vi "Create Key Map Primitive.vi"(8 "error in (no error)":errorcluster, 10 "Tresholds":refnum<class "1D Array s32.lvclass">, 11 "Keys":refnum<class "2D Array u32.lvclass">) -> (0 "error out":errorcluster, 2 "Transposed Key MapPrimitive":refnum<class "2D Array u32.lvclass">, 3 "Key Map Primitive":refnum<class "2D Array u32.lvclass">)   [LabVIEW 2020, in "G2CPU Line Profile.lvlib"]
uses:
  G2CPU Line Profile.lvlib
  <vilib>/Natan Biesmans/G2CPU GPU and CPU HPC Toolkit/G2CPU Libraries/Arrays/2DArray/u32/2D Array u32.lvclass
  C:/Program Files/National Instruments/LabVIEW 2025/vi.lib/Natan Biesmans/G2CPU GPU and CPU HPC Toolkit/G2CPU Libraries/Arrays/Array/Array Prototype.lvclass
  <vilib>/Natan Biesmans/G2CPU GPU and CPU HPC Toolkit/G2CPU Libraries/Arrays/1DArray/s32/1D Array s32.lvclass
  <vilib>/Natan Biesmans/G2CPU GPU and CPU HPC Toolkit/G2CPU Libraries/Arrays/Array/Array Prototype.lvclass/Array Prototype.ctl
  daf23bf8-e52c-43be-bfb4-cc53f6bf3ee7.vi
  0c1c3f1f-f4ad-4570-8330-175240ddfc48.vi
  daf23bf8-e52c-43be-bfb4-cc53f6bf3ee7.vi/cfed8f62-9c64-4dab-912e-5e7c21cb720b.vi
  <vilib>/Natan Biesmans/G2CPU GPU and CPU HPC Toolkit/G2CPU Libraries/Arrays/Array/G2CPU Get Array Pointer.vi
  0c1c3f1f-f4ad-4570-8330-175240ddfc48.vi/e9bebd79-1c27-4fc1-b91f-30516104c7f0.vi
  daf23bf8-e52c-43be-bfb4-cc53f6bf3ee7.vi/cfed8f62-9c64-4dab-912e-5e7c21cb720b.vi/05d18bb3-ccb1-4903-96b5-cccd48a65483.vi
  <vilib>/Natan Biesmans/G2CPU GPU and CPU HPC Toolkit/ArrayFire Driver/VIs/Run as Multi Device.vi
  daf23bf8-e52c-43be-bfb4-cc53f6bf3ee7.vi/cfed8f62-9c64-4dab-912e-5e7c21cb720b.vi/05d18bb3-ccb1-4903-96b5-cccd48a65483.vi/313ec8c5-c203-475c-9de0-0583f6fb8b4d.vi
  <vilib>/Natan Biesmans/G2CPU GPU and CPU HPC Toolkit/ArrayFire Driver/subvi/Error Converter (ErrCode or Status).vi
  <vilib>/Natan Biesmans/G2CPU GPU and CPU HPC Toolkit/G2CPU Libraries/Arrays/Array/G2CPU Set Array Pointer.vi
  <vilib>/Natan Biesmans/G2CPU GPU and CPU HPC Toolkit/ArrayFire Driver/VIs/transpose.vi
  <vilib>/Natan Biesmans/G2CPU GPU and CPU HPC Toolkit/G2CPU Libraries/Arrays/Array/G2CPU Release Array.vi
  <vilib>/Natan Biesmans/G2CPU GPU and CPU HPC Toolkit/G2CPU Libraries/Arrays/Array/Array Prototype.lvclass
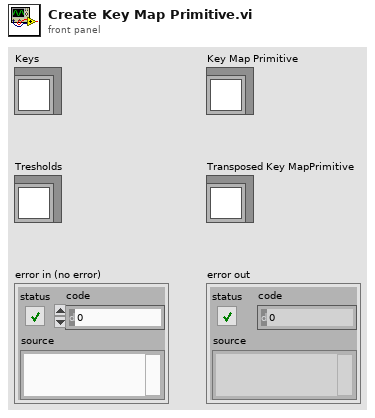
[diagram p1: front panel]
types:
  T1 = typedef "AF.lvlib/Dim4.ctl" = cluster{"Dim 0":u64, "Dim 1":u64, "Dim 2":u64, "Dim 3":u64}
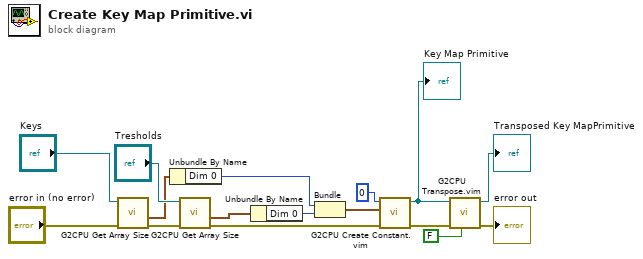
[diagram p0: block diagram]
diagram:
  n1 = call <vilib>:"G2CPU Get Array Size.vi"("error in (no error)"="error in (no error)", "Array in"="Keys") -> ("error out"=w2:errorcluster, "Array Size"=w4:T1)  [unwired: 6 in, 2 out]
  n2 = Unbundle By Name(w4) -> ("Dim 0"=w5:u64)
  n3 = call <vilib>:"G2CPU Get Array Size.vi"("error in (no error)"=w2, "Array in"="Tresholds") -> ("error out"=w13:errorcluster, "Array Size"=w6:T1)  [unwired: 6 in, 2 out]
  n4 = Unbundle By Name(w6) -> ("Dim 0"=w7:u64)
  n5 = Bundle("Dim 0"=w5, "Dim 0"=w7) -> (w3:cluster{"Dim 0":u64, "Dim 0":u64})  [unwired: 1 in]
  n6 = call "G2CPU Create Constant.vim"("error in (no error)"=w13, "Size"=w3, "val"=u32 0) -> ("error out"=w15:errorcluster, "object out"=w11:refnum<class "2D Array u32.lvclass">)  [unwired: 7 in]
  "Key Map Primitive" <- w11
  n7 = call "G2CPU Transpose.vim"("Auto Release (Enabled)"=FALSE ("Auto Release rhs (Enabled)"), "error in (no error)"=w15, "Array In"=w11) -> ("error out"=→"error out":errorcluster, "Array out"=→"Transposed Key MapPrimitive":refnum<class "2D Array u32.lvclass">)  [unwired: 7 in]
